vi "Static_3D_OBJ.vi"(6 "STL  5":path=path "C:/Users/rsKite/Desktop/stl knob files/switchstl.STL", 8 "STL 4":path=path "C:/Users/rsKite/Desktop/stl knob files/knob handlestl.STL", 9 "STL 3":path=path "C:/Users/rsKite/Desktop/stl knob files/assemstl - screwDK2-2.STL", 10 "STL 2":path=path "C:/Users/rsKite/Desktop/stl knob files/assemstl - screwDK2-1.STL", 11 "STL 1":path=path "C:/Users/rsKite/Desktop/stl knob files/assemstl - knob-1.STL") -> (1 "Child 2":refnum<vi>, 2 "Child 3":refnum<vi>, 3 "SceneObject out":refnum<vi>, 4 "Child":refnum<vi>)   [LabVIEW 2020]
uses:
  <vilib>/picture/3D Picture Control/Object/Create Object (name).vi
  <vilib>/picture/3D Picture Control/NI_3D Picture Control.lvlib
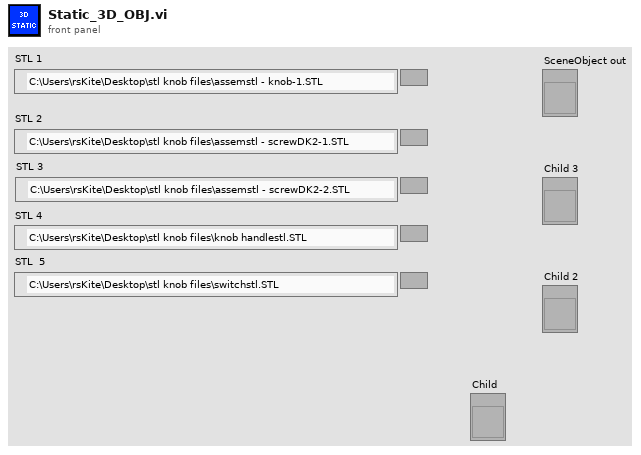
[diagram p1: front panel]
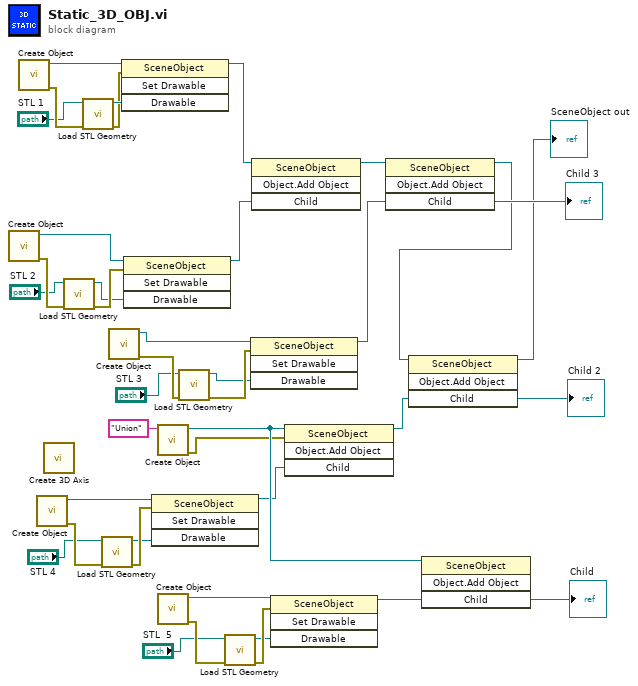
[diagram p0: block diagram]
diagram:
  n1 = call-poly <vilib>:"Create Object.vi"() -> ("error out"=w6:errorcluster, "Scene:New Object"=w10:refnum<vi>)  [unwired: 10 in]
  n2 = call-poly <vilib>:"Create Object.vi"() -> ("error out"=w3:errorcluster, "Scene:New Object"=w1:refnum<vi>)  [unwired: 10 in]
  n3 = call-poly <vilib>:"Create Object.vi"() -> ("error out"=w30:errorcluster, "Scene:New Object"=w22:refnum<vi>)  [unwired: 10 in]
  n4 = call <vilib>:"Create 3D Axis.vi"() -> ()  [unwired: 10 in, 2 out]
  n5 = call <vilib>:"Load STL Geometry.vi"("error in (no error)"=w6, "Model File"="STL 2") -> ("error out"=w9:errorcluster, "New Mesh Refnum"=w7:refnum<vi>)  [unwired: 8 in]
  n6 = call <vilib>:"Load STL Geometry.vi"("error in (no error)"=w3, "Model File"="STL 1") -> ("error out"=w4:errorcluster, "New Mesh Refnum"=w8:refnum<vi>)  [unwired: 8 in]
  n7 = call <vilib>:"Load STL Geometry.vi"("error in (no error)"=w30, "Model File"="STL 4") -> ("error out"=w24:errorcluster, "New Mesh Refnum"=w23:refnum<vi>)  [unwired: 8 in]
  n8 = call-poly <vilib>:"Create Object.vi"() -> ("error out"=w17:errorcluster, "Scene:New Object"=w14:refnum<vi>)  [unwired: 10 in]
  n9 = invoke class="SceneObject" method="Set Drawable"(reference=w1, error in=w4, "Drawable"=w8) -> (reference out=w11:refnum<vi>)  [unwired: 1 in, 3 out]
  n10 = invoke class="SceneObject" method="Set Drawable"(reference=w10, error in=w9, "Drawable"=w7) -> (reference out=w12:refnum<vi>)  [unwired: 1 in, 3 out]
  n11 = invoke class="SceneObject" method="Set Drawable"(reference=w22, error in=w24, "Drawable"=w23) -> (reference out=w31:refnum<vi>)  [unwired: 1 in, 3 out]
  n12 = call-poly <vilib>:"Create Object.vi"("Name"="Union") -> ("error out"=w32:errorcluster, "Scene:New Object"=w33:refnum<vi>)  [unwired: 9 in]
  n13 = call-poly <vilib>:"Create Object.vi"() -> ("error out"=w28:errorcluster, "Scene:New Object"=w26:refnum<vi>)  [unwired: 10 in]
  n14 = call <vilib>:"Load STL Geometry.vi"("error in (no error)"=w17, "Model File"="STL 3") -> ("error out"=w16:errorcluster, "New Mesh Refnum"=w15:refnum<vi>)  [unwired: 8 in]
  n15 = call <vilib>:"Load STL Geometry.vi"("error in (no error)"=w28, "Model File"="STL  5") -> ("error out"=w29:errorcluster, "New Mesh Refnum"=w27:refnum<vi>)  [unwired: 8 in]
  n16 = invoke class="SceneObject" method="Set Drawable"(reference=w14, error in=w16, "Drawable"=w15) -> (reference out=w19:refnum<vi>)  [unwired: 1 in, 3 out]
  n17 = invoke class="SceneObject" method="Object.Add Object"(reference=w11, "Child"=w12) -> (reference out=w18:refnum<vi>)  [unwired: 2 in, 3 out]
  n18 = invoke class="SceneObject" method="Set Drawable"(reference=w26, error in=w29, "Drawable"=w27) -> (reference out=w34:refnum<vi>)  [unwired: 1 in, 3 out]
  n19 = invoke class="SceneObject" method="Object.Add Object"(reference=w33, error in=w32, "Child"=w31) -> (reference out=w36:refnum<vi>)  [unwired: 1 in, 3 out]
  n20 = invoke class="SceneObject" method="Object.Add Object"(reference=w18, "Child"=w19) -> (reference out=w35:refnum<vi>, "Child"=→"Child 3":refnum<vi>)  [unwired: 2 in, 2 out]
  n21 = invoke class="SceneObject" method="Object.Add Object"(reference=w35, "Child"=w36) -> (reference out=→"SceneObject out":refnum<vi>, "Child"=→"Child 2":refnum<vi>)  [unwired: 2 in, 2 out]
  n22 = invoke class="SceneObject" method="Object.Add Object"(reference=w33, "Child"=w34) -> ("Child"=→"Child":refnum<vi>)  [unwired: 2 in, 3 out]
